vi "Ratio to Octaves Enum.vi"(11 "ratio":dbl=2.0) -> (3 "octaves":T1(ring)=enum."1")   [LabVIEW 2017, in "Octave with Cursors.xctl"]
uses:
  <vilib>/addons/_XControls/Octave with Cursors/Octave with Cursors.xctl
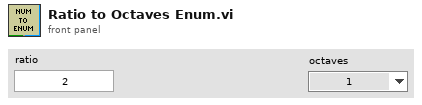
[diagram p1: front panel]
types:
  T1 = enum16{"Free", "1/24", "1/12", "1/6", "1/3", "1", "2", "4", "6", "8", "10"}
  T2 = enum16{"Free", "1/24", "1/12", "1/6", "1/3", "1", "2", "4", "6", "8", "10"}[]
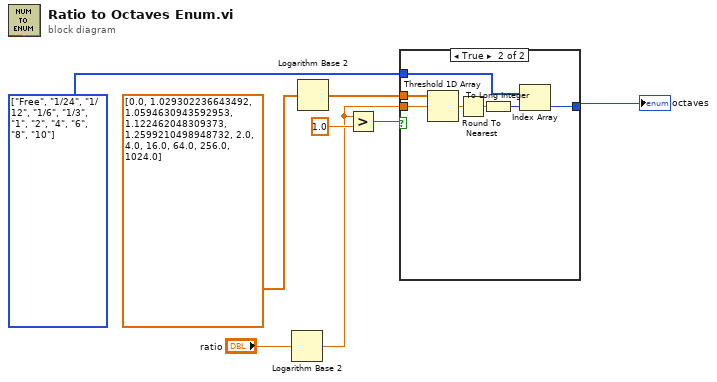
[diagram p0: block diagram]
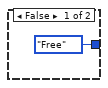
[diagram p2: hidden frame]
diagram:
  w4 = T2 [enum."Free", enum."1/24", enum."1/12", enum."1/6", enum."1/3", enum."1", enum."2", enum."4", enum."6", enum."8", enum."10"] items=["Free", "1/24", "1/12", "1/6", "1/3", "1", "2", "4", "6", "8", "10"]
  n1 = Logarithm Base 2(1:"ratio") -> (0:w1:dbl)
  n2 = Logarithm Base 2(1:dbl[] [0.0, 1.029302236643492, 1.0594630943592953, 1.122462048309373, 1.2599210498948732, 2.0, 4.0, 16.0, 64.0, 256.0, 1024.0] ("Array")) -> (0:w2:dbl[])
  n3 = Greater?(x=w1, y=1.0) -> (0:w5:bool)
  n4 = case shown="True" w5 {
    tunnel: w2 -> [_ w16]
    tunnel: w1 -> [_ w15]
    tunnel: w4 -> [_ w13]
    tunnel: [T1."Free" ("octaves") w10] -> w3
    frame False {
    }
    frame True {
      n5 = Threshold 1D Array(2:w15, 3:w16) -> (0:w14:dbl)  [unwired: 1 in]
      n6 = Round To Nearest(number=w14) -> (nearest integer value=w12:dbl)
      n7 = To Long Integer(number=w12) -> (32bit integer=w11:i32)
      n8 = Index Array(array=w13, index=w11) -> (element=w10:T1)
    }
  }
  "octaves" <- w3
